vi "Close Multi-pattern Matcher.vi"(8 "error in (no error)":errorcluster, 11 "MultiPattern Matcher in":refnum<class "MultiPattern Matcher.lvclass">) -> (0 "error out":errorcluster)   [LabVIEW 2013, in "MultiPattern Matcher.lvclass"]
uses:
  MultiPattern Matcher.lvclass
  MultiPattern Matcher.lvclass/MultiPattern Matcher.ctl
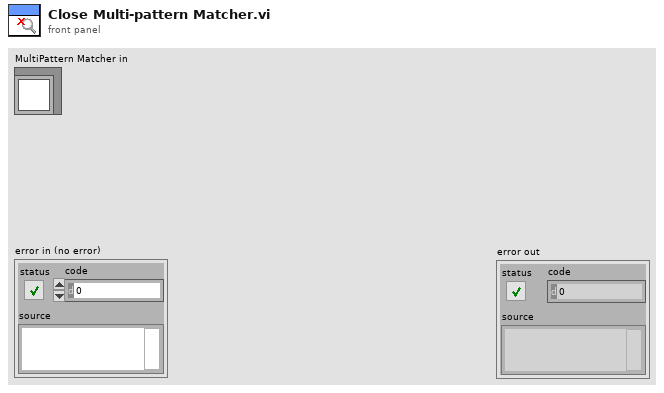
[diagram p1: front panel]
types:
  T1 = typedef "IMAQ Image.ctl" = refnum<image>
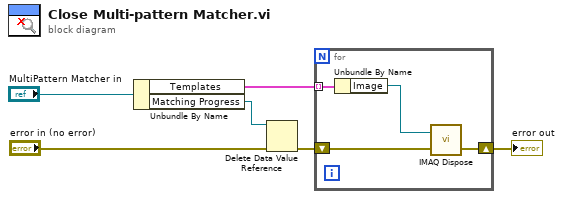
[diagram p0: block diagram]
diagram:
  n1 = Unbundle By Name("MultiPattern Matcher in") -> ("Templates"=w2:cluster{"Image":T1, "Name":string}[], "Matching Progress"=w4:refnum<data-value>)
  n2 = Delete Data Value Reference(data value reference=w4, error in="error in (no error)") -> (error out=w3:errorcluster)  [unwired: 1 out]
  n3 = for {
    shift-right: [w8] -> w1
    shift-left: w3 -> [w9]
    tunnel: w2 -> [w10] mode=indexing
    n4 = Unbundle By Name(w10) -> ("Image"=w7:T1)
    n5 = call "IMAQ Dispose"("Image"=w7, "error in (no error)"=w9) -> ("error out"=w8:errorcluster)  [unwired: 4 in]
  }
  "error out" <- w1
